vi "FTW-Setup.vi"() -> ()   [LabVIEW 2015]
panel:
  out "stderr":string
  out "stdout":string
  out "error out":errorcluster
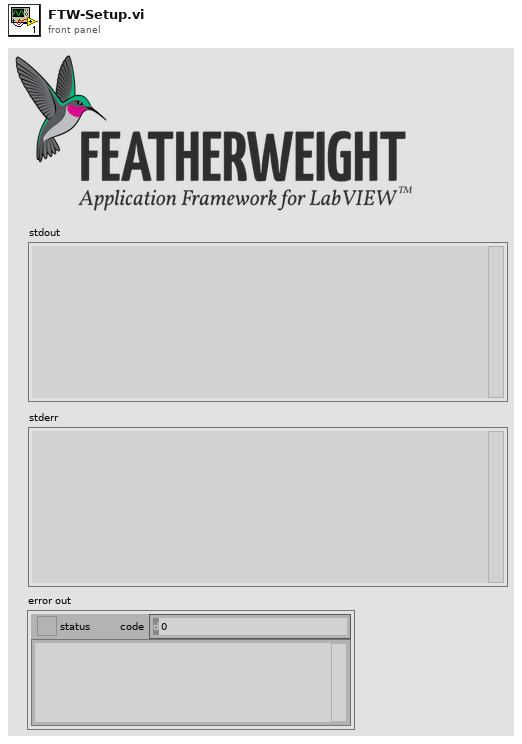
[diagram p1: front panel]
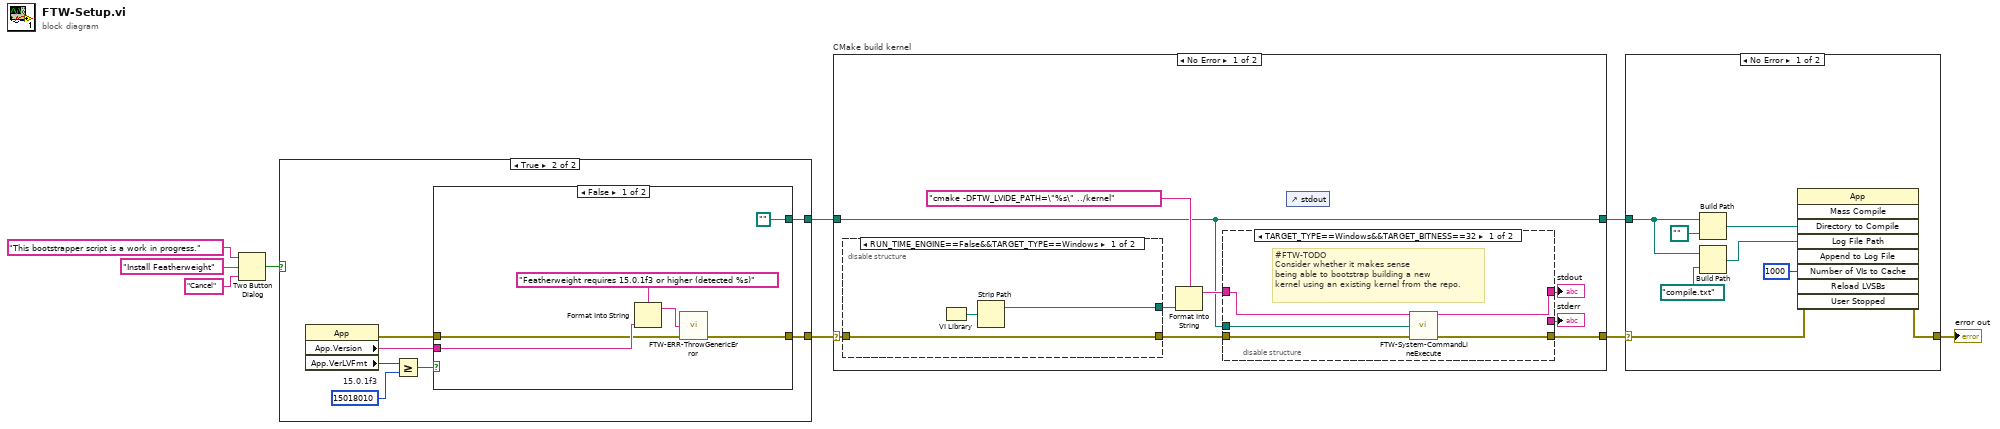
[diagram p0: block diagram]
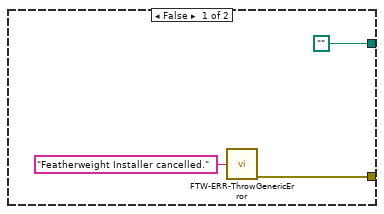
[diagram p2: hidden frame]
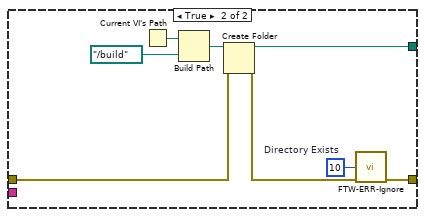
[diagram p3: hidden frame]
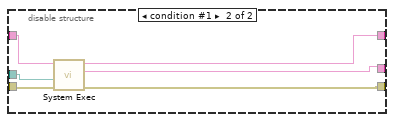
[diagram p4: hidden frame]
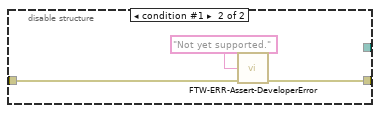
[diagram p5: hidden frame]
diagram:
  n1 = Two Button Dialog(message="This bootstrapper script is a work in progress.", 1:"Cancel" ("T button name (\"OK\")"), 2:"Install Featherweight" ("T button name (\"OK\")")) -> (T button?=w4:bool)
  n2 = case shown="True" w4 {
    tunnel: [w11 w15] -> w7
    tunnel: [path "" w13] -> w6
    frame False {
      n3 = call "FTW-ERR-ThrowGenericError.vi"("Error Message"="Featherweight Installer cancelled.") -> ("error out"=w11:errorcluster)  [unwired: 14 in]
    }
    frame True {
      w18 = 15018010  # 15.0.1f3
      n4 = property class="App"() -> (error out=w14:errorcluster, "App.Version"=w16:string, "App.VerLVFmt"=w19:i32)  [unwired: 2 in, 1 out]
      n5 = Greater Or Equal?(x=w19, y=w18) -> (x >= y?=w17:bool)
      n6 = case shown="False" w17 {
        tunnel: w16 -> [w24 _]
        tunnel: [w20 w26] -> w15
        tunnel: w14 -> [w21 w27]
        tunnel: [path "" w30] -> w13
        frame False {
          n7 = Format Into String(format string="Featherweight requires 15.0.1f3 or higher (detected %s)", w24) -> (resulting string=w22:string)  [unwired: 2 in, 1 out]
          n8 = call "FTW-ERR-ThrowGenericError.vi"("Error Message"=w22, "error in"=w21) -> ("error out"=w20:errorcluster)  [unwired: 13 in]
        }
        frame True {
          w29 = 10  # Directory Exists
          n9 = Current VI's Path() -> (path=w33:path)
          n10 = Build Path(base path=w33, name or relative path=path "../build" ("stripped path")) -> (appended path=w31:path)
          n11 = Create Folder(path (use dialog)=w31, error in=w27) -> (created path=w30:path, error out=w28:errorcluster)  [unwired: 1 in, 1 out]
          n12 = call "FTW-ERR-Ignore.vi"("Error Code"=w29, "error in"=w28) -> ("error out"=w26:errorcluster)  [unwired: 12 in, 1 out]
        }
      }
    }
  }
  n13 = case "CMake build kernel" shown="No Error" w7 {
    selector: w7 -> [w42 w61]
    tunnel: [w37 w61] -> w9
    tunnel: w6 -> [w36 w60]
    tunnel: [w36 w60] -> w3
    frame No Error {
      n14 = disable-structure shown="RUN_TIME_ENGINE==False&&TARGET_TYPE==Windows" {
        disable-tunnel: [w56 w58] -> w38
        disable-tunnel: w42 -> [w56 w59]
        disable-tunnel: [w55 _] -> w41
        frame condition #0 (active) {
          n15 = VI Library() -> (path=w54:path)
          n16 = Strip Path(path=w54) -> (stripped path=w55:path)  [unwired: 1 out]
        }
        frame condition #1 {
          n17 = call "FTW-ERR-Assert-DeveloperError.vi"("Reason this error should never happen"="Not yet supported.", "error in"=w59) -> ("error out"=w58:errorcluster)  [unwired: 13 in]
        }
      }
      n18 = Format Into String(format string="cmake -DFTW_LVIDE_PATH=\"%s\" ../kernel" ("command line"), w41) -> (resulting string=w39:string)  [unwired: 2 in, 1 out]
      n19 = disable-structure shown="TARGET_TYPE==Windows&&TARGET_BITNESS==32" {
        disable-tunnel: w39 -> [w47 w53]
        disable-tunnel: w38 -> [w46 w51]
        disable-tunnel: [w45 w50] -> w37
        disable-tunnel: w36 -> [w44 w52]
        disable-tunnel: [_ w48] -> w35
        disable-tunnel: [w43 w49] -> w34
        frame condition #0 (active) {
          # "#FTW-TODO\nConsider whether it makes sense\nbeing able to bootstrap building a new\nkernel using an existing kernel from the repo."
          n20 = call "FTW-System-CommandLineExecute.vi"("Command"=w47, "Working Directory"=w44, "error in"=w46) -> ("stdout"=w43:string, "error out"=w45:errorcluster)  [unwired: 11 in]
        }
        frame condition #1 {
          n21 = call <vilib>:"System Exec.vi"("error in (no error)"=w51, "working directory"=w52, "command line"=w53) -> ("error out"=w50:errorcluster, "standard error"=w48:string, "standard output"=w49:string)  [unwired: 5 in, 1 out]
        }
      }
      "stderr" <- w35
      "stdout" <- w34
      n22 = control-ref of="stdout"() -> ()  [unwired: 1 out]
    }
    frame Error {
    }
  }
  n23 = case shown="No Error" w9 {
    selector: w9 -> [w66 w70]
    tunnel: [w65 w70] -> w8
    tunnel: w3 -> [w62 _]
    frame No Error {
      n24 = Build Path(base path=w62, name or relative path=path ".." ("stripped path")) -> (appended path=w63:path)
      n25 = Build Path(base path=w62, name or relative path=path "compile.txt" ("stripped path")) -> (appended path=w68:path)
      n26 = invoke class="App" method="Mass Compile"(error in=w66, "Directory to Compile"=w63, "Log File Path"=w68, "Number of VIs to Cache"=u32 1000) -> (error out=w65:errorcluster)  [unwired: 5 in, 8 out]
    }
    frame Error {
    }
  }
  "error out" <- w8
